vi "SSM2603 Read Register.vi"(8 "Error In (No Error)":errorcluster, 10 "Reg Address":u8, 11 "FPGA VI Reference In":T1) -> (0 "error out":errorcluster, 2 "Reg Data":i16 format="b%09b", 3 "FPGA VI Reference Out":T1)   [LabVIEW 2015]
uses:
  DSDB FPGA Ref.ctl
panel:
  # "Overview: This VI use I2C to read SSM2603 registers. SSM2603 use 9-bit registers to configure chip."
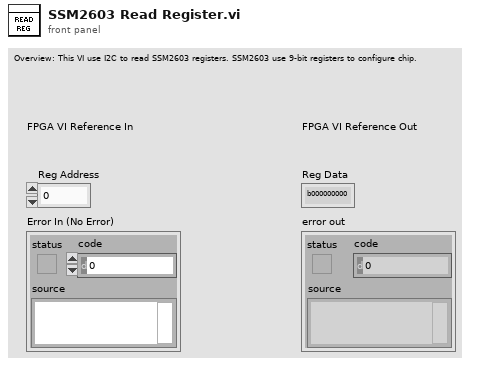
[diagram p1: front panel]
types:
  T1 = typedef "DSDB FPGA Ref.ctl" = refnum<k20>
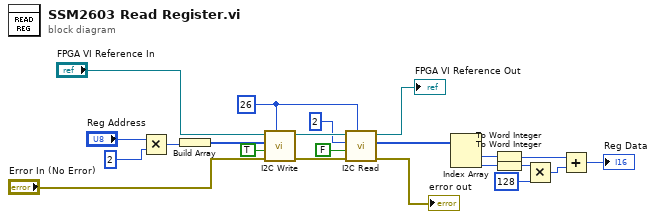
[diagram p0: block diagram]
diagram:
  w19 = u8 26 ("Slave Address (7-bit)")
  n1 = Multiply(x="Reg Address", y=u8 2) -> (x*y=w14:u8)
  n2 = Build Array(w14) -> (w13:u8[])
  n3 = call "I2C Write.vi"("Slave Address (7-bit)"=w19, "Error In (No Error)"="Error In (No Error)", "Keep Bus Busy"=TRUE, "Data to Write"=w13, "FPGA VI Reference In"="FPGA VI Reference In") -> ("error out"=w20:errorcluster, "FPGA VI Reference Out"=w21:T1)  [unwired: 5 in]
  n4 = call "I2C Read.vi"("Slave Address (7-bit)"=w19, "Error In (No Error)"=w20, "Keep Bus Busy"=FALSE, "Bytes to Read"=u32 2, "FPGA VI Reference In"=w21) -> ("error out"=→"error out":errorcluster, "Data Read"=w8:u8[], "FPGA VI Reference Out"=→"FPGA VI Reference Out":T1)  [unwired: 4 in]
  n5 = Index Array(array=w8) -> (element #1=w7:u8, element #2=w6:u8)  [unwired: 2 in]
  n6 = To Word Integer(number=w7) -> (16bit integer=w2:i16)
  n7 = To Word Integer(number=w6) -> (16bit integer=w5:i16)
  n8 = Multiply(x=w5, y=i16 128) -> (x*y=w3:i16)
  n9 = Add(x=w2, y=w3) -> (x+y=→"Reg Data":i16)
